vi "_Build query command substring.vi"(0 "System no.":i32=1 min=1 max=4 step=1, 2 "Axes to query in":string[](array[string]), 3 "Query\nAll axes?":bool, 4 "For all axes: use\nAxis identifier?":bool=TRUE, 6 "With space?":bool) -> (14 "Command substring":string, 15 "Axes to query out":string[](array[string]), 16 "Number of rows":u32=1)   [LabVIEW 2019]
doc: "This VI builds a query command substring. If All axes is TRUE, connected axes are read from \"Global2.vi\" and returned in Axes to query out, otherwise Axes to query out is identical with Axes to query in. Number of rows is size of the Axes to query out array. If Axis identifier is FALSE, command substring is an empty string (e.c. for systems which accept commands like POS? without axis IDs). If \"With space?\" is true or system supports GCS 2.0, a space character is added between the axes identifiers.\nExample: If axes A;B;C;D are connected to the system to command, Axes to query in is A;B;D, Query all axes? is TRUE and Use Axis identifier is TRUE, resulting Command substring is \"ABCD\", Number of rows is 4 and Axes to query out is A;B;C;D.\n\nValid for all systems"
panel:
  # "This vi builds a query command substring. If \"Query all axes\" is true, connected axes are read from\nGlobal2.vi. If \"Use axis identifier\" is false, command substring is an empty string (e.c. for POS?). If\n\"With space?\" is true or system supports GCS 2.0, a space character is added between the axes identifiers."
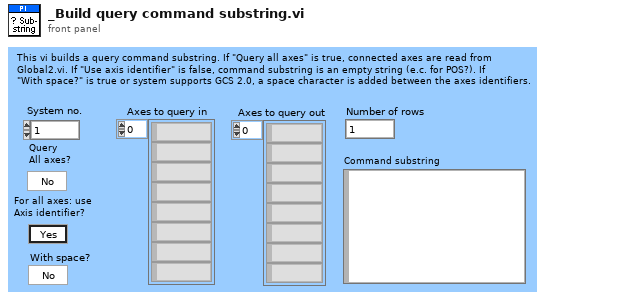
[diagram p1: front panel]
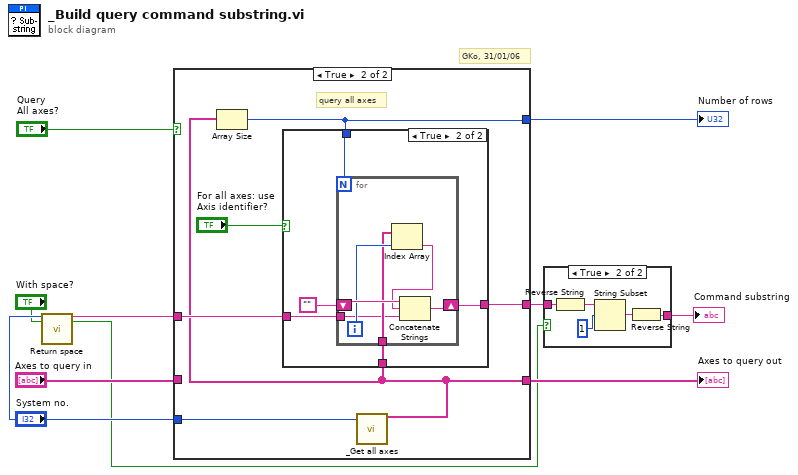
[diagram p0: block diagram]
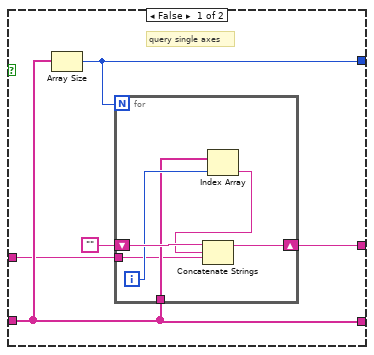
[diagram p3: hidden frame]
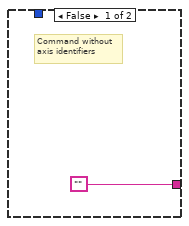
[diagram p4: hidden frame]
diagram:
  # "GKo, 31/01/06"
  n1 = call "Return space.vi"("System no."="System no.", "With space?"="With space?") -> ("String out"=w1:string, "Space returned?"=w3:bool)  [unwired: 16 in]
  n2 = case shown="True" "Query\nAll axes?" {
    tunnel: [w14 w27] -> w5
    tunnel: "Axes to query in" -> [w13 _]
    tunnel: [w13 w23] -> w7
    tunnel: [w12 w26] -> w10
    tunnel: w1 -> [w11 w24]
    tunnel: "System no." -> [_ w22]
    frame False {
      # "query single axes"
      n3 = Array Size(array=w13) -> (size(s)=w12:i32)
      n4 = for {
        N: w12 -> [_]
        shift-right: [w20] -> w14
        shift-left: "" -> [w21]
        tunnel: w13 -> [w17]
        tunnel: w11 -> [w16]
        i -> [w19]
        n5 = Index Array(array=w17, index=w19) -> (element=w18:string)
        n6 = Concatenate Strings(w21, w18, w16) -> (w20:string)
      }
    }
    frame True {
      # "query all axes"
      n7 = call "_Get all axes.vi"("System no."=w22) -> ("Conn. Axes"=w23:string[])  [unwired: 18 in]
      n8 = Array Size(array=w23) -> (size(s)=w26:i32)
      n9 = case shown="True" "For all axes: use\nAxis identifier?" {
        tunnel: ["" w30] -> w27
        tunnel: w23 -> [_ w33]
        tunnel: w26 -> [_ w31]
        tunnel: w24 -> [_ w29]
        frame False {
          # "Command without\naxis identifiers"
        }
        frame True {
          n10 = for {
            N: w31 -> [_]
            shift-right: [w38] -> w30
            shift-left: "" -> [w39]
            tunnel: w33 -> [w35]
            tunnel: w29 -> [w34]
            i -> [w37]
            n11 = Index Array(array=w35, index=w37) -> (element=w36:string)
            n12 = Concatenate Strings(w39, w36, w34) -> (w38:string)
          }
        }
      }
    }
  }
  "Number of rows" <- w10
  "Axes to query out" <- w7
  n13 = case shown="True" w3 {
    tunnel: [w40 w41] -> w6
    tunnel: w5 -> [w40 w43]
    frame False {
    }
    frame True {
      n14 = Reverse String(1:w43) -> (0:w45:string)
      n15 = String Subset(string=w45, offset (0)=1) -> (substring=w42:string)  [unwired: 1 in]
      n16 = Reverse String(1:w42) -> (0:w41:string)
    }
  }
  "Command substring" <- w6
